vi "SPV.vi"(0 "System no.":i32=1 min=1 max=4 step=1, 1 "Target Memory Type":T1, 2 "ContainerUnit":string, 3 "FunctionUnit":string, 4 "ParameterID":string, 5 "error in":errorcluster, 6 "Value":string) -> (19 "error out":errorcluster)   [LabVIEW 2020]
doc: "SPV (Set Parameter Value)\n\nDescription\nSets the value for a Configuration parameter (p. 119) in a memory of the controller.\n\nFormat\nSPV <MemType> <Container Unit> <Function Unit> <ParameterID> <Value>\n\nArguments\nThe available Configuration parameters and their properties (including <Container Unit>, \n<Function Unit>, <ParameterID>, dimension of the parameter, data type and range for the \nparameter value) can be queried with the USG? PAM command (p. 77). \n<MemType>\nType of memory in which the value is to be set\nPossible values: RAM, TMP, FLASH\n<Container Unit>\nContainer unit, whose parameter is to be set\nPossible values: Alias of the container unit (p. 94) \n<Function Unit>\nFunction unit, whose parameter is to be set\nIf a parameter belonging to a container unit is to be set, \"-\" must be entered for <Function \nUnit>.\nPossible values:\nAlias of the function unit (p. 94) \n\"-\" \n<ParameterID>\nThe value of the parameter addressed by <Container Unit>, <Function Unit> and <ParameterID> \nwill be set in the specified memory.\n<ParameterID> always contains a parameter identifier in hexadecimal format. For 0-\ndimensional parameters, <ParameterID> is fully specified by the parameter identifier.\nFor one-dimensional and multi-dimensional parameters, an element address is also required \ntogether with the parameter identifier. Depending on the dimension of the parameter, the \nelement address consists of one or more parts that are separated from the parameter identifier \nand each other by a comma.\n- One-dimensional parameter (vector) ? the element address is ,number\n- Two-dimensional parameter (two-dimensional matrix) ? the element address is \n,number,number\n- Three-dimensional parameter (three-dimensional matrix) ? the element address \nis ,number,number,number\nThe address data for the parameters can be queried with USG? PAM (p. 77). \nPossible values:\n0x0000 to 0xFFFF\nFor one-dimensional and multi-dimensional parameters, an additional integer = 1 for each \ndimension\n<Value>\nParameter value\nPossible values: Dependent on the parameter\n\nResponse\nnone\n\nExample\nThe P term of the PID controller is to be set immediately to the value 100 for axis 1 in the \nworking memory of the controller. Beforehand, the current values for all parameters of the PID\ncontroller for axis 1 are queried in the working memory.\nNote: The user command level (p. 69) for write access to the parameter is \"ADV\" (see <WRITEUCL> in the response to USG? PAM). Therefore, it is necessary to change to this user command \nlevel before setting the parameter.\n>>spv? ram axis_1 cntr_1\n<<RAM AXIS_1 CNTR_1 0x101=0.0\n<<RAM AXIS_1 CNTR_1 0x102=0.0\n<<RAM AXIS_1 CNTR_1 0x103=0\n<<RAM AXIS_1 CNTR_1 0x104=0.0\n<<RAM AXIS_1 CNTR_1 0x105=1.0\n<<RAM AXIS_1 CNTR_1 0x110=0\n<<RAM AXIS_1 CNTR_1 0x111=10.0E-3 \n<<RAM AXIS_1 CNTR_1 0x112=50.0E-3 \n<<RAM AXIS_1 CNTR_1 0x113=0\n<<RAM AXIS_1 CNTR_1 0x120,1=50.0\n<<RAM AXIS_1 CNTR_1 0x121,1=75.0E-3 \n<<RAM AXIS_1 CNTR_1 0x122,1=0\n<<RAM AXIS_1 CNTR_1 0x123=1\n<<RAM AXIS_1 CNTR_1 0x124,1=10000.0\n>>ucl?\n<<USR\n>>ucl adv advanced\n>>ucl?\n<<ADV\n>>spv ram axis_1 cntr_1 0x120,1 100\n>>spv? ram axis_1 cntr_1 0x120,1\n<<RAM AXIS_1 CNTR_1 0x120,1=100.0\n>>err?\n<<0 - (error 0 - \"No error\")\n\nNotes\nThe response to USG? PAM includes the user command level for write access (<WRITE-UCL> \ncolumn) to the parameter value. The UCL? command (p. 71) queries the active user command \nlevel. Use the UCL command (p. 69) to change to the appropriate user command level.\nThe value of a parameter can be read from the different memories of the controller using the \nSPV? command (p. 63). \nThe CPA command (p. 8) can be used to copy the values of configuration parameters between \nthe different memories of the controller.\nFor further details, see \"Parameter Handling - GCS 3.0\" (p. 119). \n\nUser command level\nUSR"
uses:
  ConfigurationMemoryType.ctl
panel:
  # "SPV (Set Parameter Value)\n\nSets the value for a Configuration parameter in a memory of the controller."
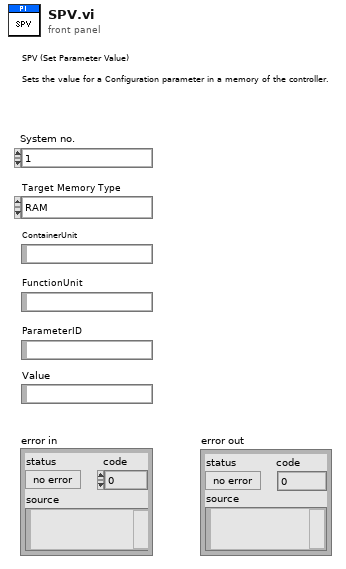
[diagram p1: front panel]
types:
  T1 = typedef "ConfigurationMemoryType.ctl" = enum16{"RAM", "TMP", "FLASH"}
  T2 = typedef "Syntax.ctl" = enum16{"GCS 1.0", "GCS 2.0", "GCS 3.0"}
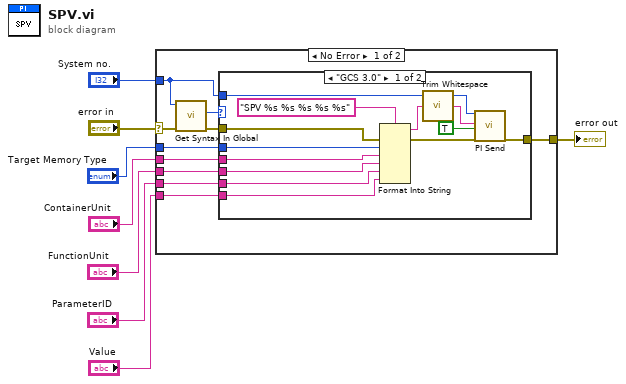
[diagram p0: block diagram]
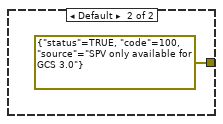
[diagram p2: hidden frame]
diagram:
  n1 = case shown="No Error" "error in" {
    selector: "error in" -> [w16 w33]
    tunnel: [w15 w33] -> w7
    tunnel: "System no." -> [w14 _]
    tunnel: "ParameterID" -> [w10 _]
    tunnel: "Target Memory Type" -> [w13 _]
    tunnel: "FunctionUnit" -> [w11 _]
    tunnel: "ContainerUnit" -> [w12 _]
    tunnel: "Value" -> [w9 _]
    frame No Error {
      n2 = call "Get Syntax In Global.vi"("error in"=w16, "System no."=w14) -> ("error out"=w18:errorcluster, "Syntax"=w17:T2)  [unwired: 8 in]
      n3 = case shown="\"GCS 3.0\"" w17 {
        tunnel: [w25 errorcluster {"status"=TRUE, "code"=100, "source"="SPV only available for GCS 3.0"} ("error out")] -> w15
        tunnel: w18 -> [w27 _]
        tunnel: w14 -> [w24 _]
        tunnel: w13 -> [w23 _]
        tunnel: w12 -> [w22 _]
        tunnel: w11 -> [w21 _]
        tunnel: w10 -> [w20 _]
        tunnel: w9 -> [w19 _]
        frame "GCS 3.0" {
          n4 = Format Into String(format string="SPV %s %s %s %s %s", error in=w27, w23, w22, w21, w20, w19) -> (resulting string=w29:string, error out=w26:errorcluster)  [unwired: 1 in]
          n5 = call <vilib>:"Trim Whitespace.vi"("string"=w29) -> ("trimmed string"=w30:string)  [unwired: 1 in]
          n6 = call "PI Send.vi"("System no."=w24, "String to send"=w30, "Attach termination char.?"=TRUE, "error in"=w26) -> ("error out"=w25:errorcluster)  [unwired: 2 in, 13 out]
        }
        frame Default {
        }
      }
    }
    frame Error {
    }
  }
  "error out" <- w7
